vi "test.vi"() -> ()   [LabVIEW 2015]
panel:
  in  "stop":bool
  out "Numeric":i32
  in  "Slide":dbl(slide) scale=0.0..10.0
  out "Array 2":i32[](array[numeric])
  out "output array":i32[][](array[numeric])
  out "Array":i32[](array[numeric])
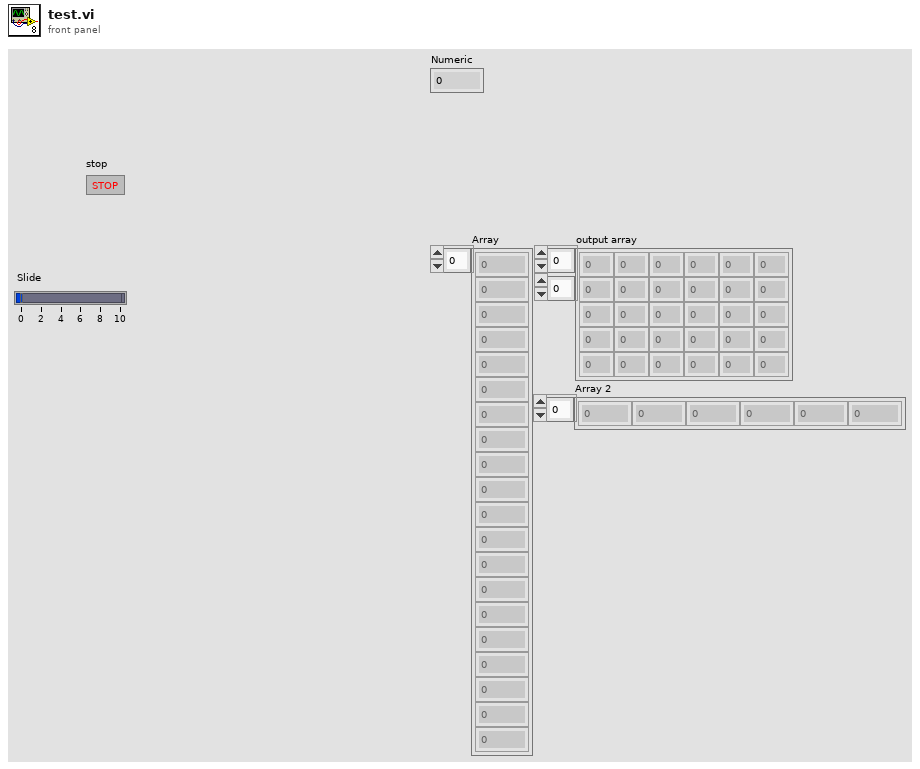
[diagram p1: front panel]
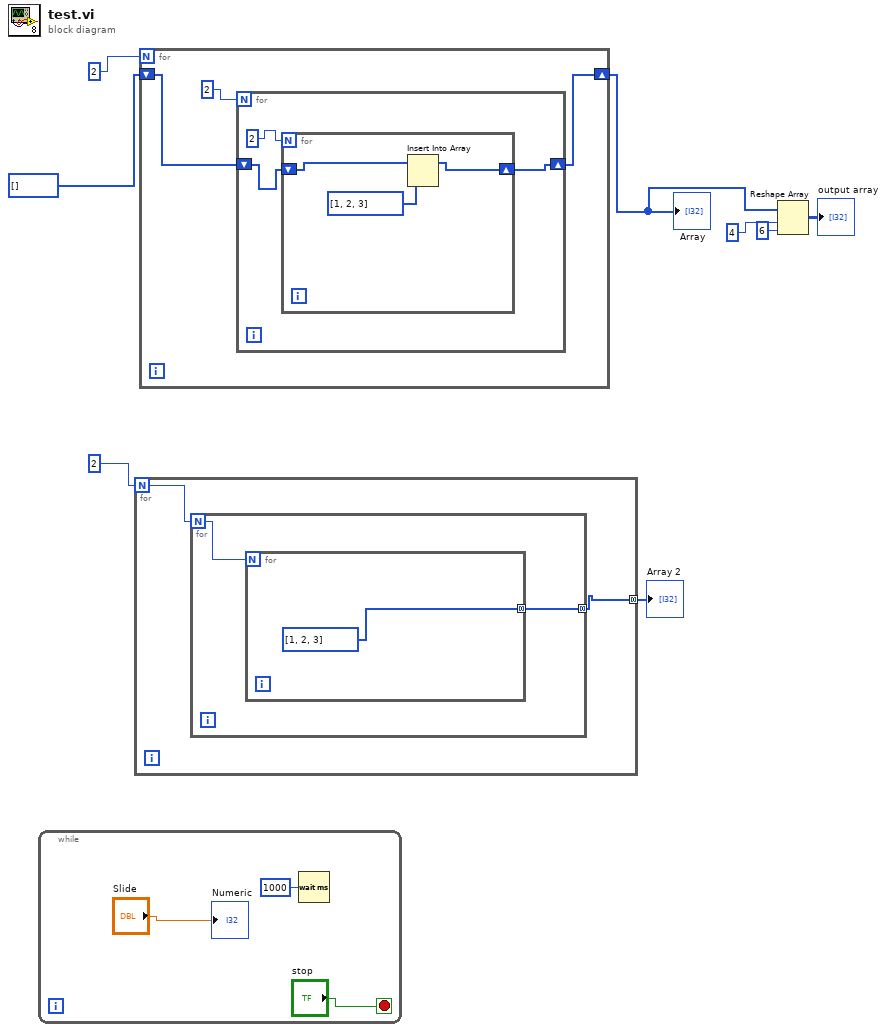
[diagram p0: block diagram]
diagram:
  n1 = while {
    stop <- "stop" stop-if-true
    n2 = Wait (ms)(milliseconds to wait=u32 1000) -> ()  [unwired: 1 out]
    "Numeric" <- "Slide"
  }
  n3 = for {
    N: 2 -> [w12]
    tunnel: [w13] -> w2 mode=concatenating
    n4 = for {
      N: w12 -> [w14]
      tunnel: [w15] -> w13 mode=concatenating
      n5 = for {
        N: w14 -> [_]
        tunnel: [i32[] [1, 2, 3]] -> w15 mode=concatenating
      }
    }
  }
  "Array 2" <- w2
  n6 = for {
    N: 2 -> [_]
    shift-right: [w17] -> w6
    shift-left: i32[] [] -> [w18]
    n7 = for {
      N: 2 -> [_]
      shift-right: [w20] -> w17
      shift-left: w18 -> [w21]
      n8 = for {
        N: 2 -> [_]
        shift-right: [w24] -> w20
        shift-left: w21 -> [w25]
        n9 = Insert Into Array(array=w25, new element=i32[] [1, 2, 3]) -> (w24:i32[])  [unwired: 1 in]
      }
    }
  }
  "Array" <- w6
  n10 = Reshape Array(w6, 4, 6 ("dimension size")) -> (→"output array":i32[][])
